vi "SerialMoveZ.vi"(2 "error in (no error)":errorcluster, 4 "Z":i32, 5 "baud rate (9600)":u32=9600) -> (0 "error out":errorcluster)   [LabVIEW 2010]
doc: "Establishes connection with configured port (default = COM1).\nSends command MOVE X=x Y=y where x and y are integers denoting 10ths of a micron.\nSub-VI SerialWaitForStatusN.vi polls controller with STATUS command until 'N' (not busy) status is returned, or until a configured maximum number of unsuccessful tries (default = 400).\nDisconnects from configured port."
uses:
  <vilib>/Instr/_visa.llb/VISA Configure Serial Port (Instr).vi
  Instance           1 19Saved   SerialMoveZ .vi
panel:
  out "resulting string":string
  out "Success":bool
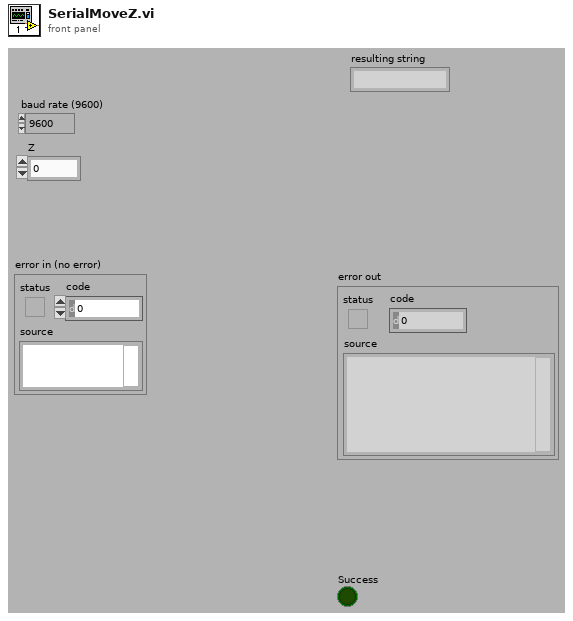
[diagram p1: front panel]
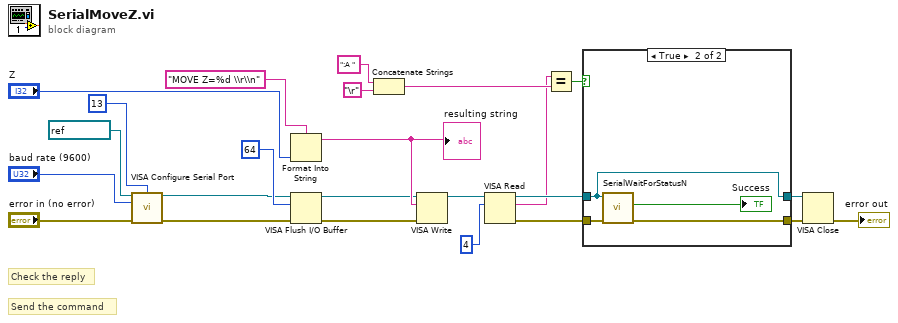
[diagram p0: block diagram]
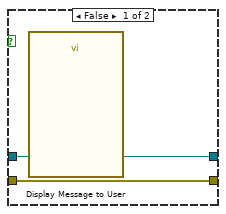
[diagram p2: hidden frame]
diagram:
  # "Check the reply"
  # "Send the command"
  n1 = call-poly "VISA Configure Serial Port"("VISA resource name"=refnum<visa-resource-name> "COM3", "termination char\n(0xA = '\\n' = LF)"=u8 13 ("termination char\n(0xA = '\\n' = LF)"), "baud rate (9600)"="baud rate (9600)", "error in (no error)"="error in (no error)") -> ("VISA resource name out"=w7:refnum<visa-resource-name>, "error out"=w5:errorcluster)  [unwired: 3 in, 7 out]
  n2 = Format Into String "Format Into String"(format string="MOVE Z=%d \\r\\n", "Z") -> (resulting string=w14:string)  [unwired: 2 in, 1 out]
  "resulting string" <- w14
  n3 = VISA Flush I/O Buffer(VISA resource name=w7, mask (16)=u16 64, error in (no error)=w5) -> (VISA resource name out=w10:refnum<visa-resource-name>, error out=w9:errorcluster)
  n4 = Concatenate Strings "Concatenate Strings"(":A " ("y"), "\r") -> (w22:string)
  n5 = VISA Write(VISA resource name=w10, write buffer=w14, error in (no error)=w9) -> (VISA resource name out=w24:refnum<visa-resource-name>)  [unwired: 2 out]
  n6 = VISA Read(VISA resource name=w24, byte count=u32 4) -> (VISA resource name out=w18:refnum<visa-resource-name>, read buffer=w12:string, error out=w17:errorcluster)  [unwired: 1 in, 1 out]
  n7 = Equal?(x=w12, y=w22) -> (x = y?=w19:bool)
  n8 = case shown="True" w19 {
    tunnel: w18 -> [w25 w27]
    tunnel: w17 -> [w26 w30]
    tunnel: [w26 w29] -> w13
    tunnel: [w25 w27] -> w2
    frame False {
      n9 = call "Display Message to User"() -> ()  [unwired: 3 in, 9 out]
    }
    frame True {
      n10 = call "SerialWaitForStatusN.vi"("error out 2"=w30, "VISA resource name(COM1)"=w27) -> ("error out"=w29:errorcluster, "Success"=→"Success":bool)  [unwired: 3 in, 2 out]
    }
  }
  n11 = VISA Close(VISA resource name=w2, error in (no error)=w13) -> (error out=→"error out":errorcluster)
